vi "Write DataMap.vi"(8 "error in (no error)":errorcluster, 10 "DataMap":refnum<data-value>, 11 "Exe Write Main CMD in":refnum<class "Exe Write PAS Wvfm CMD.lvclass">) -> (0 "error out":errorcluster, 3 "Exe Write Main CMD out":refnum<class "Exe Write PAS Wvfm CMD.lvclass">)   [LabVIEW 2018, in "Controller.lvlib" / "Exe Write PAS Wvfm CMD.lvclass"]
uses:
  Exe Write PAS Wvfm CMD.lvclass
  Exe Write PAS Wvfm CMD.lvclass/Exe Write PAS Wvfm CMD.ctl
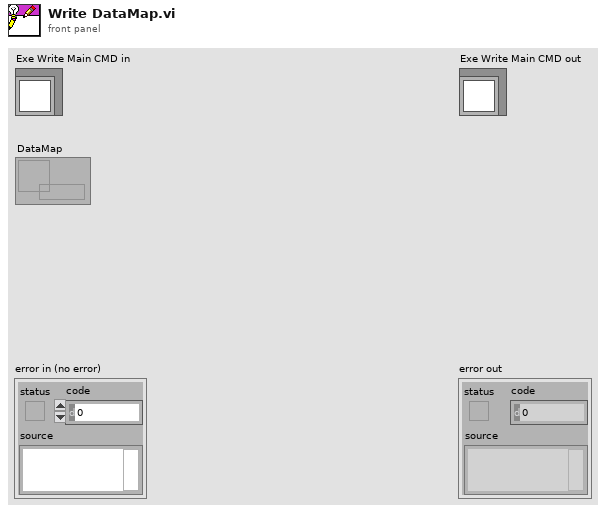
[diagram p1: front panel]
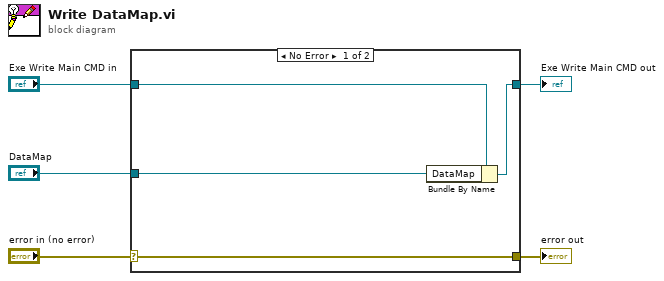
[diagram p0: block diagram]
diagram:
  n1 = case shown="No Error" "error in (no error)" {
    selector: "error in (no error)" -> [w9 w10]
    tunnel: [w9 w10] -> w4
    tunnel: [w7 w11] -> w2
    tunnel: "Exe Write Main CMD in" -> [w8 w11]
    tunnel: "DataMap" -> [w6 _]
    frame No Error {
      n2 = Bundle By Name(cluster=w8, "DataMap"=w6) -> (w7:refnum<class "Exe Write PAS Wvfm CMD.lvclass">)
    }
    frame Error {
    }
  }
  "error out" <- w4
  "Exe Write Main CMD out" <- w2
